vi "assign_id.vi"() -> ()   [LabVIEW 2015]
uses:
  <vilib>/MakerHub/LINX/Public/Utilities/Open Serial.vi
  <vilib>/MakerHub/LINX/LMH-LINX.lvlib
panel:
  in  "Device User ID 2":u16
  out "Device User ID":u16
  out "Error Out":errorcluster
  in  "Serial Port":refnum<visa-resource-name>="N/A"
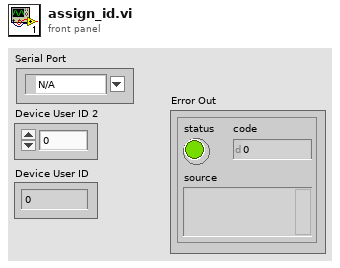
[diagram p1: front panel]
types:
  T1 = typedef "LMH-LINX.lvlib/LINX Ref.ctl" = cluster{"IO":T2, "Interface":T3, "LINX Device Config":T4}
  T2 = typedef "LMH-LINX.lvlib/Platform.ctl" = enum16{"Remote", "Local"}
  T3 = typedef "LMH-LINX.lvlib/Interface.ctl" = enum16{"Serial", "TCP"}
  T4 = typedef "LMH-LINX.lvlib/Device.lvlib/LINX Device Config.ctl" = cluster{"Interface":T3, "COM Port":refnum<visa-resource-name>, "TCP Configuration":T5, "Device Family":u8, "Device ID":u8, "Device Name":string, "TCP Ref":refnum<k5>, "Channels":T6}
  T5 = typedef "LMH-LINX.lvlib/Device.lvlib/TCP Config.ctl" = cluster{"IP Address":string, "Port":u16}
  T6 = typedef "LMH-LINX.lvlib/Channels.ctl" = cluster{"DI":u8[], "DO":u8[], "AI":u8[], "AO":u8[], "PWM":u8[], "QE":u8[], "UART":u8[], "I2C 2":u8[], "SPI":u8[], "CAN":u8[], "Servo":u8[], "AI Ref (V)":dbl, "AI Resolution (Bits)":u8, "AO Ref (V)":dbl, "AO Resolution (Bits)":u8}
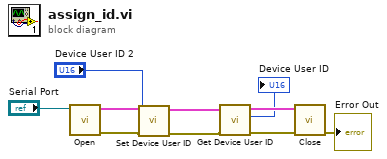
[diagram p0: block diagram]
diagram:
  n1 = call-poly <vilib>:"Open.vi"("Serial Port"="Serial Port") -> ("Error Out"=w2:errorcluster, "LINX Resource"=w5:T1)  [unwired: 8 in, 1 out]
  n2 = call <vilib>:"Set Device User ID.vi"("Error In"=w2, "Device User ID"="Device User ID 2", "LINX Resource"=w5) -> ("Error Out"=w3:errorcluster, "LINX Resource"=w4:T1)  [unwired: 7 in]
  n3 = call <vilib>:"Get Device User ID.vi"("Error In"=w3, "LINX Resource"=w4) -> ("Error Out"=w8:errorcluster, "Device User ID"=→"Device User ID":u16, "LINX Resource"=w9:T1)  [unwired: 7 in]
  n4 = call <vilib>:"Close.vi"("Error In"=w8, "LINX Resource"=w9) -> ("Error Out"=→"Error Out":errorcluster)  [unwired: 9 in]
